vi "Write Invert Action.vi"(10 "Invert Action":bool, 11 "Valve in":refnum<class "Valve.lvclass">) -> (3 "Valve out":refnum<class "Valve.lvclass">)   [LabVIEW 2015, in "cRIO-Carbondioxide.lvlib" / "CO2-Actor.lvlib" / "Valve.lvclass"]
uses:
  Valve.lvclass
  Valve.lvclass/Valve.ctl
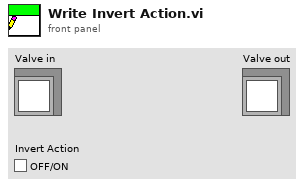
[diagram p1: front panel]
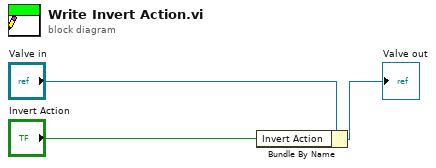
[diagram p0: block diagram]
diagram:
  n1 = Bundle By Name(cluster="Valve in", "Invert Action"="Invert Action") -> (→"Valve out":refnum<class "Valve.lvclass">)
